vi "AuMT8852B Test Parameter.vi"(0 "VISA session":refnum<visa-resource-name>, 1 "Test (Output power)":T2(ring), 2 "Parameter (Use low frequency)":T1, 3 "Range check? (F)":bool, 4 "Simulate? (F)":bool, 5 "error in (no error)":errorcluster, 6 "Set/Get (Set)":enum16{"Set", "Get"}(ring), 8 "Script (3)":i32=3, 10 "Integer value (0)":i32, 12 "Float value (0)":dbl format="%.2f") -> (11 "Integer value out":i32, 13 "Float value out":dbl format="%.2f", 14 "VISA session out":refnum<visa-resource-name>, 19 "error out":errorcluster)   [LabVIEW 2017]
doc: "Anritsu MT8852B Bluetooth Tester\n\nWrites or reads a single test parameter from the instrument. This VI is a tool for use by higher-level configuration functions. Not all combinations of tests and parameters are valid.\n\nINPUTS\nSet/Get - whether the parameter will be sent to or received from the instrument.\nScript - test script (1-10) containing the test being configured. Scripts 1 and 2 are read-only.\nTest - type of test to be configured.\nParameter - property of the test to be read or written.\nRange check? - whether or not this VI should reject out-of-range values.\nSimulate? - whether or not this VI should skip the instrument I/O.\nInteger value - value to be written (for integer/boolean parameters).\nFloat value - value to be written (for floating-point parameters).\n\nOUTPUTS\nInteger value out - value read from instrument (for integer/boolean parameters).\nFloat value out - value read from instrument (for floating-point parameters)."
uses:
  <instrlib>/aumt8852B/General/Utilities/MT8850 Test Parameters.ctl
  <instrlib>/aumt8852B/General/Utilities/MT8850 Frequency Units.ctl
panel:
  out "Response":string
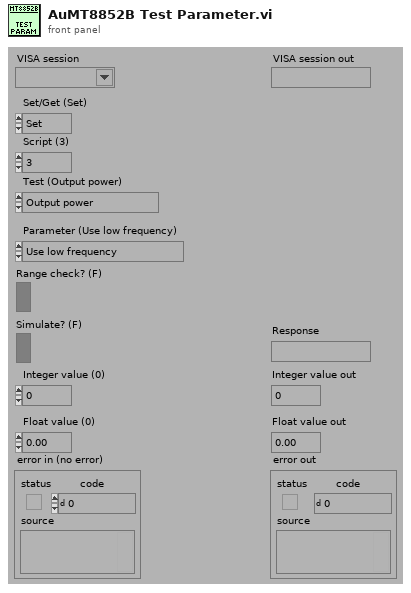
[diagram p1: front panel]
types:
  T1 = typedef "MT8850 Test Parameters.ctl" = enum16{"Use low frequency", "Use medium frequency", "Use high frequency", "Low TX frequency", "Low RX frquency", "Medium TX frequency", "Medium RX frequency", "High TX frequency", "High RX frequency", "Number of packets", "Average high limit", "Average low limit", "Peak power limit", "Max power step limit", "Min power step limit", "f1 average minimum", "f1 average maximum", "f2 maximum", "f1/f2 average maximum", "Hop selection", "Use DH1 packets", "Use DH3 packets", "Use DH5 packets", "1 slot packet drift limit", "3 slot packet drift limit", "5 slot packet drift limit", "Drift rate limit", "TX power level", "Frequency offset", "Symbol timing", "Modulation index", "BER limit", "FER limit", "Use averaging high limit", "Use averaging low limit", "Use peak power limit", "Packet type", "Test control", "Use max power step limit", "Use min power step limit", "Number of cycles", "Use f1 average maximum", "Use f1 average minimum", "Use f2 maximum", "Use f1/f2 average maximum", "Hop mode", "Maximum negative limit", "Maximum positive limit", "Use maximum negative limit", "Use maximum positive limit", "Use 1 slot packet drift limit", "Use 3 slot packet drift limit", "Use 5 slot packet drift limit", "Use drift rate limit", "Use BER limit", "Use FER limit", "Use dirty parameter table", "Use null packet drift limit", "Null packet drift limit", "Minimum power", "Power delay", "Packet count", "Payload toggle", "Output power level", "2DHX packet type", "3DHX packet type", "Number of blocks", "TX and RX low frequency", "TX and RX medium frequency", "TX and RX high frequency", "TX frequency", "RX frequency", "Threshold bit count", "Total test bit count", "Number of bits", "PDPSK to PGFSK lower limit", "PDPSK to PGFSK upper limit", "Initial frequency error upper limit", "Initial frequency error lower limit", "Frequency error upper limit", "Frequency error lower limit", "Block frequency error upper limit", "Block frequency error lower limit", "2Mbs RMS DEVM limit", "3Mbs RMS DEVM limit", "2Mbs Peak DEVM limit", "3Mbs Peak DEVM limit", "2Mbs 99% packets DEVM limit", "3Mbs 99% packets DEVM limit", "Percentage of no error packets limit", "Threshold error limit", "Total test error limit"}
  T2 = enum16{"Output power", "Power control", "Modulation characteristics", "Initial carrier", "Carrier drift", "Single slot sensitivity", "Multiple slot sensitivity", "Maximum input power"}
  T3 = typedef "MT8850 Frequency Units.ctl" = enum16{"Channel", "Hz", "kHz", "MHz", "GHz"}
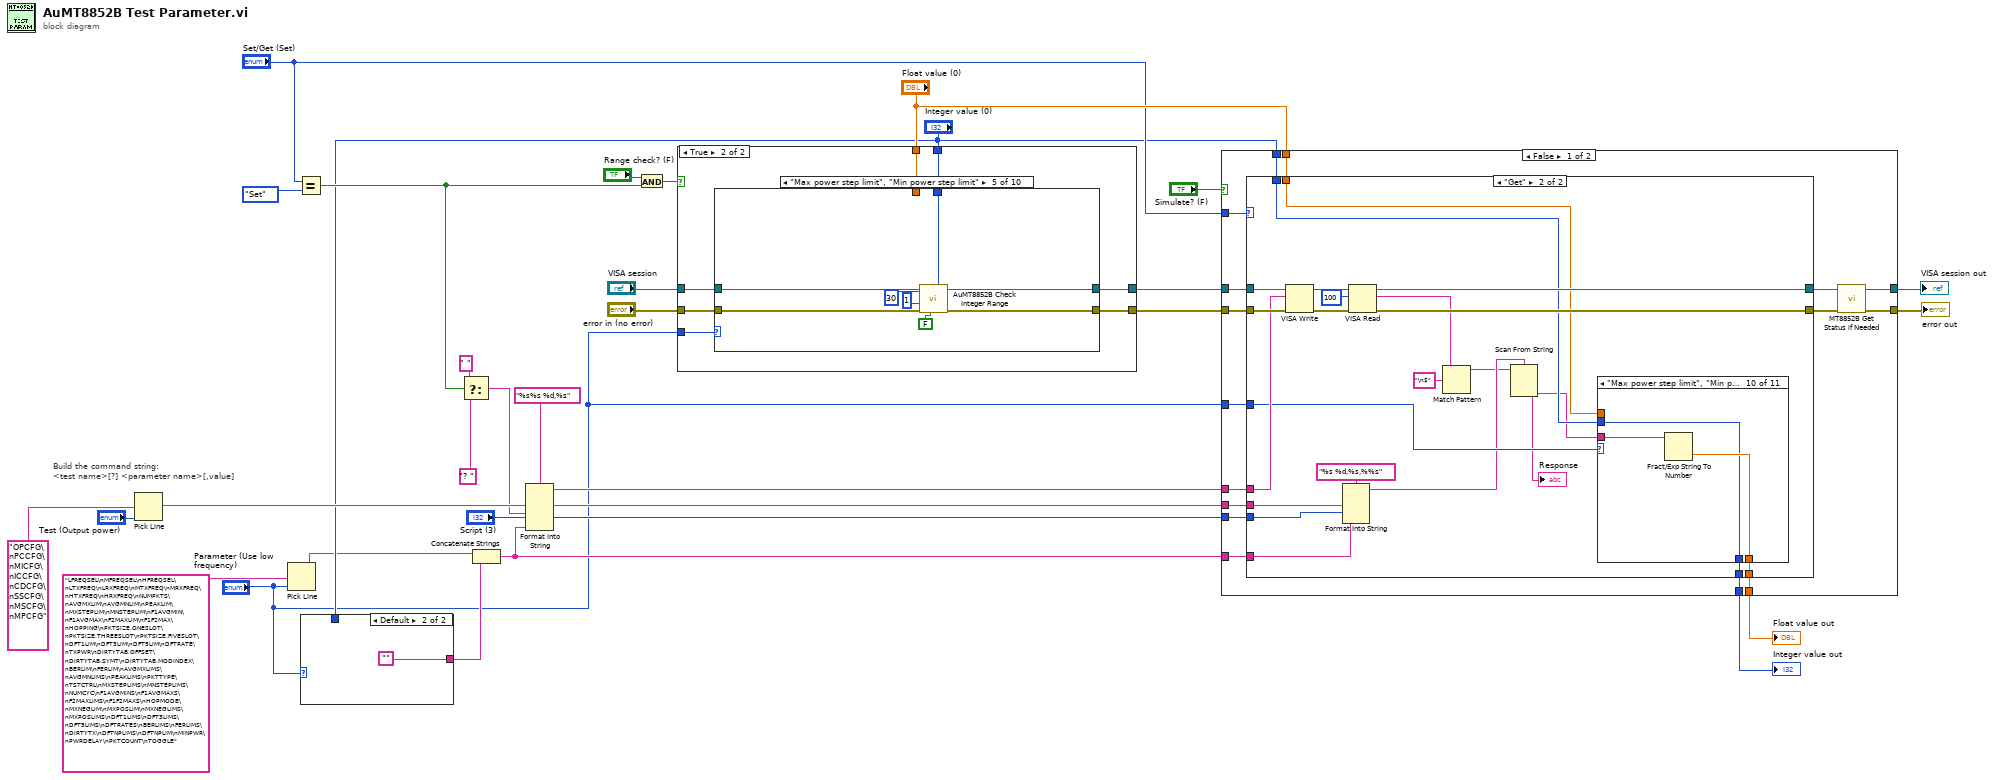
[diagram p0: block diagram]
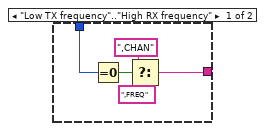
[diagram p2: hidden frame]
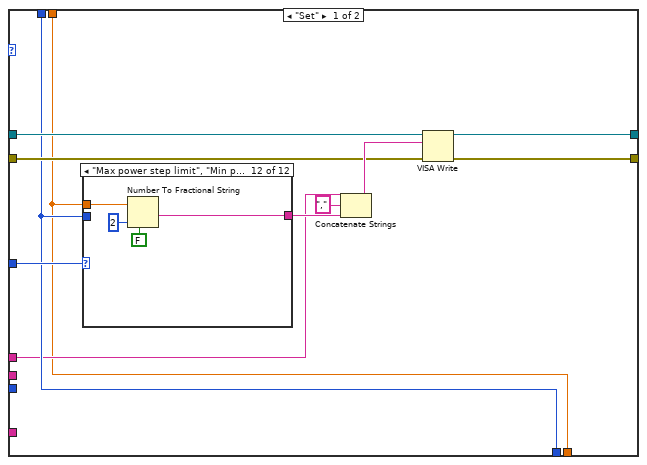
[diagram p3: hidden frame]
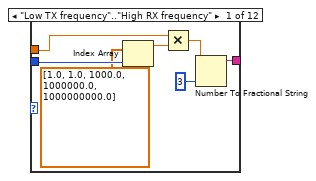
[diagram p4: hidden frame]
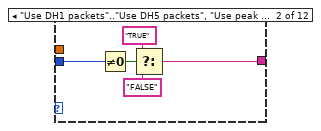
[diagram p5: hidden frame]
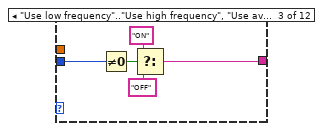
[diagram p6: hidden frame]
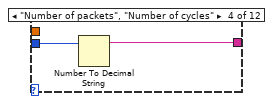
[diagram p7: hidden frame]
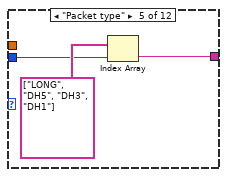
[diagram p8: hidden frame]
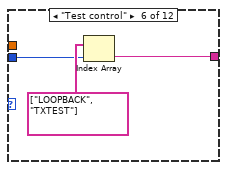
[diagram p9: hidden frame]
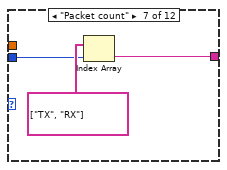
[diagram p10: hidden frame]
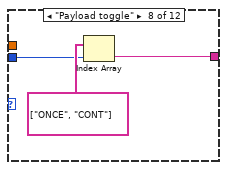
[diagram p11: hidden frame]
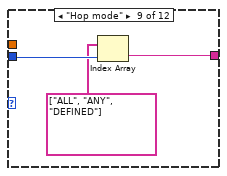
[diagram p12: hidden frame]
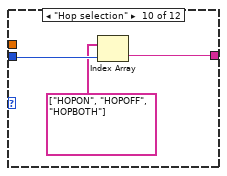
[diagram p13: hidden frame]
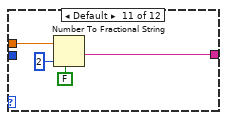
[diagram p14: hidden frame]
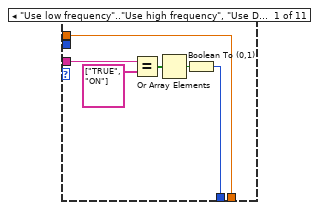
[diagram p15: hidden frame]
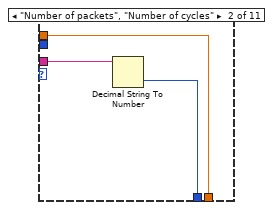
[diagram p16: hidden frame]
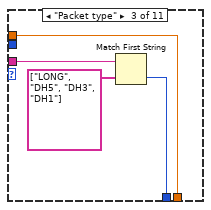
[diagram p17: hidden frame]
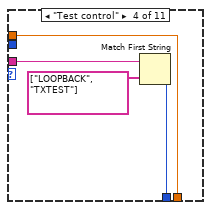
[diagram p18: hidden frame]
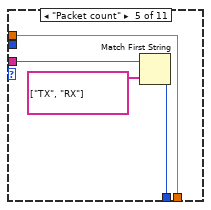
[diagram p19: hidden frame]
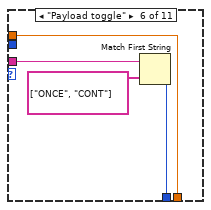
[diagram p20: hidden frame]
diagram:
  # "Build the command string:\n<test name>[?] <parameter name>[,value]"
  n1 = Pick Line(multi-line string="OPCFG\nPCCFG\nMICFG\nICCFG\nCDCFG\nSSCFG\nMSCFG\nMPCFG", line index="Test (Output power)") -> (output string=w10:string)  [unwired: 1 in]
  n2 = Pick Line(multi-line string="LFREQSEL\nMFREQSEL\nHFREQSEL\nLTXFREQ\nLRXFREQ\nMTXFREQ\nMRXFREQ\nHTXFREQ\nHRXFREQ\nNUMPKTS\nAVGMXLIM\nAVGMNLIM\nPEAKLIM\nMXSTEPLIM\nMNSTEPLIM\nF1AVGMIN\nF1AVGMAX\nF2MAXLIM\nF1F2MAX\nHOPPING\nPKTSIZE,ONESLOT\nPKTSIZE,THREESLOT\nPKTSIZE,FIVESLOT\nDFT1LIM\nDFT3LIM\nDFT5LIM\nDFTRATE\nTXPWR\nDIRTYTAB,OFFSET\nDIRTYTAB,SYMT\nDIRTYTAB,MODINDEX\nBERLIM\nFERLIM\nAVGMXLIMS\nAVGMNLIMS\nPEAKLIMS\nPKTTYPE\nTSTCTRL\nMXSTEPLIMS\nMNSTEPLIMS\nNUMCYC\nF1AVGMINS\nF1AVGMAXS\nF2MAXLIMS\nF1F2MAXS\nHOPMODE\nMXNEGLIM\nMXPOSLIM\nMXNEGLIMS\nMXPOSLIMS\nDFT1LIMS\nDFT3LIMS\nDFT5LIMS\nDFTRATES\nBERLIMS\nFERLIMS\nDIRTYTX\nDFTNPLIMS\nDFTNPLIM\nMINPWR\nPWRDELAY\nPKTCOUNT\nTOGGLE", line index="Parameter (Use low frequency)") -> (output string=w4:string)  [unwired: 1 in]
  n3 = Equal?(x="Set/Get (Set)", y=enum16{"Set", "Get"}."Set") -> (x = y?=w20:bool)
  n4 = case shown="Default" "Parameter (Use low frequency)" {
    tunnel: "Integer value (0)" -> [w35 _]
    tunnel: [w31 ""] -> w3
    frame "Low TX frequency".."High RX frequency" {
      n5 = Equal To 0?(x=w35) -> (x = 0?=w34:bool)
      n6 = Select(t=",CHAN" ("Substring"), s=w34, f=",FREQ" ("Substring")) -> (s? t:f=w31:string)
    }
    frame Default {
    }
  }
  n7 = Select(t=" ", s=w20, f="? ") -> (s? t:f=w9:string)
  n8 = Concatenate Strings(w4, w3) -> (w5:string)
  n9 = Format Into String(format string="%s%s %d,%s" ("Format String"), w10, w9, "Script (3)", w5) -> (resulting string=w2:string)  [unwired: 2 in, 1 out]
  n10 = And(x="Range check? (F)", y=w20) -> (x .and. y?=w22:bool)
  n11 = case shown="True" w22 {
    tunnel: "Parameter (Use low frequency)" -> [_ w45]
    tunnel: "Integer value (0)" -> [_ w44]
    tunnel: "Float value (0)" -> [_ w43]
    tunnel: "VISA session" -> [w38 w42]
    tunnel: "error in (no error)" -> [w37 w41]
    tunnel: [w38 w40] -> w17
    tunnel: [w37 w39] -> w16
    frame False {
    }
    frame True {
      n12 = case shown="\"Max power step limit\", \"Min power step limit\"" w45 {
        tunnel: w44 -> [_ w50 w75 _ w87 _ _ _ _ _]
        tunnel: w43 -> [_ w48 _ w84 _ w95 w103 w111 w119 w127]
        tunnel: w42 -> [w47 w56 w72 w80 w89 w97 w105 w113 w121 w129]
        tunnel: w41 -> [w46 w55 w71 w79 w88 w96 w104 w112 w120 w128]
        tunnel: [w47 w58 w70 w78 w86 w94 w102 w110 w118 w126] -> w40
        tunnel: [w46 w57 w69 w77 w85 w93 w101 w109 w117 w125] -> w39
        frame Default {
        }
        frame "Low TX frequency".."High RX frequency" {
          n13 = Type Cast(type=MT8850_Frequency_Units."MHz" ("Frequency units (MHz)"), x=w50) -> (*(type *) &x=w51:T3)
          n14 = case shown="\"Channel\"" w51 {
            tunnel: [78.0 2480000000.0 2480000.0 2480.0 2.48] -> w54
            tunnel: [0.0 2402000000.0 2402000.0 2402.0 2.402] -> w53
            frame "Channel" {
            }
            frame "Hz" {
            }
            frame "kHz" {
            }
            frame "MHz" {
            }
            frame "GHz" {
            }
          }
          n15 = call <instrlib>:"AuMT8852B Check Float Range.vi"("Value (0)"=w48, "Check IVI flag first? (T)"=FALSE, "error in (no error)"=w55, "Lower limit (-1)"=w53, "Upper limit (1)"=w54, "VISA session"=w56) -> ("error out"=w57:errorcluster, "VISA session out"=w58:refnum<visa-resource-name>)  [unwired: 4 in]
        }
        frame "Number of packets", "Number of cycles" {
          n16 = call <instrlib>:"AuMT8852B Check Integer Range.vi"("Value (0)"=w75, "Check IVI flag first? (T)"=FALSE, "error in (no error)"=w71, "Lower limit (-1)"=1, "Upper limit (1)"=10000, "VISA session"=w72) -> ("error out"=w69:errorcluster, "VISA session out"=w70:refnum<visa-resource-name>)  [unwired: 4 in]
        }
        frame "Average high limit".."Peak power limit" {
          n17 = call <instrlib>:"AuMT8852B Check Float Range.vi"("Value (0)"=w84, "Check IVI flag first? (T)"=FALSE, "error in (no error)"=w79, "Lower limit (-1)"=-10.0, "Upper limit (1)"=30.0, "VISA session"=w80) -> ("error out"=w77:errorcluster, "VISA session out"=w78:refnum<visa-resource-name>)  [unwired: 4 in]
        }
        frame "Max power step limit", "Min power step limit" {
          n18 = call <instrlib>:"AuMT8852B Check Integer Range.vi"("Value (0)"=w87, "Check IVI flag first? (T)"=FALSE, "error in (no error)"=w88, "Lower limit (-1)"=1, "Upper limit (1)"=30, "VISA session"=w89) -> ("error out"=w85:errorcluster, "VISA session out"=w86:refnum<visa-resource-name>)  [unwired: 4 in]
        }
        frame "Frequency offset" {
          n19 = call <instrlib>:"AuMT8852B Check Float Range.vi"("Value (0)"=w95, "Check IVI flag first? (T)"=FALSE, "error in (no error)"=w96, "Lower limit (-1)"=-75000.0, "Upper limit (1)"=75000.0, "VISA session"=w97) -> ("error out"=w93:errorcluster, "VISA session out"=w94:refnum<visa-resource-name>)  [unwired: 4 in]
        }
        frame "Symbol timing" {
          n20 = call <instrlib>:"AuMT8852B Check Float Range.vi"("Value (0)"=w103, "Check IVI flag first? (T)"=FALSE, "error in (no error)"=w104, "Lower limit (-1)"=-20.0, "Upper limit (1)"=20.0, "VISA session"=w105) -> ("error out"=w101:errorcluster, "VISA session out"=w102:refnum<visa-resource-name>)  [unwired: 4 in]
        }
        frame "Modulation index" {
          n21 = call <instrlib>:"AuMT8852B Check Float Range.vi"("Value (0)"=w111, "Check IVI flag first? (T)"=FALSE, "error in (no error)"=w112, "Lower limit (-1)"=0.25, "Upper limit (1)"=0.38, "VISA session"=w113) -> ("error out"=w109:errorcluster, "VISA session out"=w110:refnum<visa-resource-name>)  [unwired: 4 in]
        }
        frame "Minimum power" {
          n22 = call <instrlib>:"AuMT8852B Check Float Range.vi"("Value (0)"=w119, "Check IVI flag first? (T)"=FALSE, "error in (no error)"=w120, "Lower limit (-1)"=-40.0, "Upper limit (1)"=0.0, "VISA session"=w121) -> ("error out"=w117:errorcluster, "VISA session out"=w118:refnum<visa-resource-name>)  [unwired: 4 in]
        }
        frame "Power delay" {
          n23 = call <instrlib>:"AuMT8852B Check Float Range.vi"("Value (0)"=w127, "Check IVI flag first? (T)"=FALSE, "error in (no error)"=w128, "Lower limit (-1)"=0.1, "Upper limit (1)"=100.0, "VISA session"=w129) -> ("error out"=w125:errorcluster, "VISA session out"=w126:refnum<visa-resource-name>)  [unwired: 4 in]
        }
      }
    }
  }
  n24 = case shown="False" "Simulate? (F)" {
    tunnel: "Parameter (Use low frequency)" -> [w148 _]
    tunnel: "Integer value (0)" -> [w147 w275]
    tunnel: "Float value (0)" -> [w146 w274]
    tunnel: "Set/Get (Set)" -> [w145 _]
    tunnel: w2 -> [w140 _]
    tunnel: w17 -> [w144 w273]
    tunnel: w16 -> [w143 w272]
    tunnel: [w133 w273] -> w15
    tunnel: [w134 w272] -> w8
    tunnel: [w142 w275] -> w14
    tunnel: [w141 w274] -> w13
    tunnel: w10 -> [w139 _]
    tunnel: w5 -> [w138 _]
    tunnel: "Script (3)" -> [w137 _]
    frame False {
      n25 = case shown="\"Get\"" w145 {
        tunnel: w148 -> [w159 w218]
        tunnel: w147 -> [w151 w215]
        tunnel: w146 -> [w149 w214]
        tunnel: w140 -> [w150 w224]
        tunnel: w144 -> [w155 w226]
        tunnel: w143 -> [w154 w225]
        tunnel: [w153 w220] -> w136
        tunnel: [w152 w219] -> w135
        tunnel: [w151 w217] -> w142
        tunnel: [w149 w216] -> w141
        tunnel: w139 -> [_ w212]
        tunnel: w138 -> [_ w210]
        tunnel: w137 -> [_ w211]
        frame "Set" {
          n26 = case shown="\"Max power step limit\", \"Min power step limit\"" w159 {
            tunnel: w151 -> [w166 w168 w173 w178 w180 w183 w186 w189 w193 w196 _ _]
            tunnel: w149 -> [w164 _ _ _ _ _ _ _ _ _ w200 w204]
            tunnel: [w160 w167 w172 w177 w179 w182 w185 w188 w192 w195 w199 w203] -> w157
            frame "Low TX frequency".."High RX frequency" {
              n27 = Index Array(array=dbl[] [1.0, 1.0, 1000.0, 1000000.0, 1000000000.0] ("Array Constant"), index=w166) -> (element=w165:dbl)
              n28 = Multiply(x=w164, y=w165) -> (x*y=w162:dbl)
              n29 = Number To Fractional String(number=w162, precision (6)=i16 3) -> (F-format string=w160:string)  [unwired: 2 in]
            }
            frame "Use DH1 packets".."Use DH5 packets", "Use peak power limit", "Use max power step limit", "Use min power step limit", "Use f1 average maximum".."Use f1/f2 average maximum", "Use maximum negative limit".."Use FER limit" {
              n30 = Not Equal To 0?(x=w168) -> (x != 0?=w171:bool)
              n31 = Select(t="TRUE", s=w171, f="FALSE") -> (s? t:f=w167:string)
            }
            frame "Use low frequency".."Use high frequency", "Use averaging high limit", "Use averaging low limit", "Use dirty parameter table", "Use null packet drift limit" {
              n32 = Not Equal To 0?(x=w173) -> (x != 0?=w176:bool)
              n33 = Select(t="ON", s=w176, f="OFF") -> (s? t:f=w172:string)
            }
            frame "Number of packets", "Number of cycles" {
              n34 = Number To Decimal String(number=w178) -> (decimal integer string=w177:string)  [unwired: 1 in]
            }
            frame "Packet type" {
              n35 = Index Array(array=string[] ["LONG", "DH5", "DH3", "DH1"] ("Array Constant"), index=w180) -> (element=w179:string)
            }
            frame "Test control" {
              n36 = Index Array(array=string[] ["LOOPBACK", "TXTEST"] ("Array Constant"), index=w183) -> (element=w182:string)
            }
            frame "Packet count" {
              n37 = Index Array(array=string[] ["TX", "RX"] ("Array Constant"), index=w186) -> (element=w185:string)
            }
            frame "Payload toggle" {
              n38 = Index Array(array=string[] ["ONCE", "CONT"] ("Array Constant"), index=w189) -> (element=w188:string)
            }
            frame "Hop mode" {
              n39 = Index Array(array=string[] ["ALL", "ANY", "DEFINED"] ("Array Constant"), index=w193) -> (element=w192:string)
            }
            frame "Hop selection" {
              n40 = Index Array(array=string[] ["HOPON", "HOPOFF", "HOPBOTH"] ("Array Constant"), index=w196) -> (element=w195:string)
            }
            frame Default {
              n41 = Number To Fractional String(use system decimal point (T)=FALSE, number=w200, precision (6)=i16 2) -> (F-format string=w199:string)  [unwired: 1 in]
            }
            frame "Max power step limit", "Min power step limit" {
              n42 = Number To Fractional String(use system decimal point (T)=FALSE, number=w204, precision (6)=i16 2) -> (F-format string=w203:string)  [unwired: 1 in]
            }
          }
          n43 = Concatenate Strings(w150, "," ("Substring"), w157) -> (w156:string)
          n44 = VISA Write(VISA resource name=w155, write buffer=w156, error in (no error)=w154) -> (VISA resource name out=w153:refnum<visa-resource-name>, error out=w152:errorcluster)  [unwired: 1 out]
        }
        frame "Get" {
          n45 = VISA Write(VISA resource name=w226, write buffer=w224, error in (no error)=w225) -> (VISA resource name out=w223:refnum<visa-resource-name>, error out=w222:errorcluster)  [unwired: 1 out]
          n46 = Format Into String(format string="%s %d,%s,%%s" ("Format String"), w212, w211, w210) -> (resulting string=w209:string)  [unwired: 2 in, 1 out]
          n47 = VISA Read(VISA resource name=w223, byte count=u32 100 ("byte count (0)"), error in (no error)=w222) -> (VISA resource name out=w220:refnum<visa-resource-name>, read buffer=w207:string, error out=w219:errorcluster)  [unwired: 1 out]
          n48 = Match Pattern(string=w207, regular expression="\n$") -> (before substring=w205:string)  [unwired: 1 in, 3 out]
          n49 = Scan From String(format string=w209, input string=w205) -> (output 1=w208:string)  [unwired: 3 in, 3 out]
          "Response" <- w208
          n50 = case shown="\"Max power step limit\", \"Min power step limit\"" w218 {
            tunnel: w208 -> [w232 w235 w238 w242 w246 w250 w254 w258 w262 w265 w271]
            tunnel: [w231 w234 w237 w241 w245 w249 w253 w257 w260 w263 w266] -> w217
            tunnel: [w230 w233 w236 w240 w244 w248 w252 w256 w261 w264 w267] -> w216
            tunnel: w215 -> [_ _ _ _ _ _ _ _ w260 w263 w266]
            tunnel: w214 -> [w230 w233 w236 w240 w244 w248 w252 w256 _ _ _]
            frame "Use low frequency".."Use high frequency", "Use DH1 packets".."Use DH5 packets", "Use averaging high limit".."Use peak power limit", "Use max power step limit", "Use min power step limit", "Use f1 average maximum".."Use f1/f2 average maximum", "Use maximum negative limit".."Use null packet drift limit" {
              n51 = Equal?(x=w232, y=string[] ["TRUE", "ON"] ("Array Constant")) -> (x = y?=w228:bool[])
              n52 = Or Array Elements(Boolean array=w228) -> (logical OR=w227:bool)
              n53 = Boolean To (0,1)(Boolean=w227) -> (0, 1=w231:i16)
            }
            frame "Number of packets", "Number of cycles" {
              n54 = Decimal String To Number(string=w235) -> (number=w234:i32)  [unwired: 2 in, 1 out]
            }
            frame "Packet type" {
              n55 = Match First String(2:string[] ["LONG", "DH5", "DH3", "DH1"] ("Array Constant"), 3:w238) -> (0:w237:i32)  [unwired: 1 out]
            }
            frame "Test control" {
              n56 = Match First String(2:string[] ["LOOPBACK", "TXTEST"] ("Array Constant"), 3:w242) -> (0:w241:i32)  [unwired: 1 out]
            }
            frame "Packet count" {
              n57 = Match First String(2:string[] ["TX", "RX"] ("Array Constant"), 3:w246) -> (0:w245:i32)  [unwired: 1 out]
            }
            frame "Payload toggle" {
              n58 = Match First String(2:string[] ["ONCE", "CONT"] ("Array Constant"), 3:w250) -> (0:w249:i32)  [unwired: 1 out]
            }
            frame "Hop mode" {
              n59 = Match First String(2:string[] ["ALL", "ANY", "DEFINED"] ("Array Constant"), 3:w254) -> (0:w253:i32)  [unwired: 1 out]
            }
            frame "Hop selection" {
              n60 = Match First String(2:string[] ["HOPON", "HOPOFF", "HOPBOTH"] ("Array Constant"), 3:w258) -> (0:w257:i32)  [unwired: 1 out]
            }
            frame Default {
              n61 = Fract/Exp String To Number(string=w262) -> (number=w261:dbl)  [unwired: 3 in, 1 out]
            }
            frame "Max power step limit", "Min power step limit" {
              n62 = Fract/Exp String To Number(string=w265) -> (number=w264:dbl)  [unwired: 3 in, 1 out]
            }
            frame "Low TX frequency".."High RX frequency" {
              n63 = Fract/Exp String To Number(string=w271) -> (number=w269:dbl)  [unwired: 3 in, 1 out]
              n64 = Index Array(array=dbl[] [1.0, 1.0, 1000.0, 1000000.0, 1000000000.0] ("Array Constant"), index=w266) -> (element=w268:dbl)
              n65 = Divide(x=w269, y=w268) -> (x/y=w267:dbl)
            }
          }
        }
      }
      n66 = call <instrlib>:"MT8852B Get Status if Needed.vi"("error in (no error)"=w135, "VISA session"=w136) -> ("error out"=w134:errorcluster, "VISA session out"=w133:refnum<visa-resource-name>)  [unwired: 8 in]
    }
    frame True {
    }
  }
  "VISA session out" <- w15
  "error out" <- w8
  "Integer value out" <- w14
  "Float value out" <- w13
